vi "Ref_Num_Stopwatch_CapTest.vi"(4 "Elapsed time (seconds)":refnum<vi>, 5 "start time":refnum<vi>, 6 "stop":refnum<vi>, 7 "OK Button":refnum<vi>, 11 "Started":refnum<vi>) -> ()   [LabVIEW 2020]
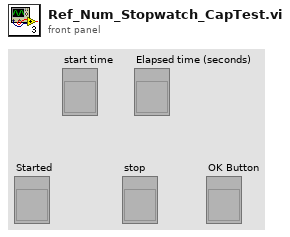
[diagram p1: front panel]
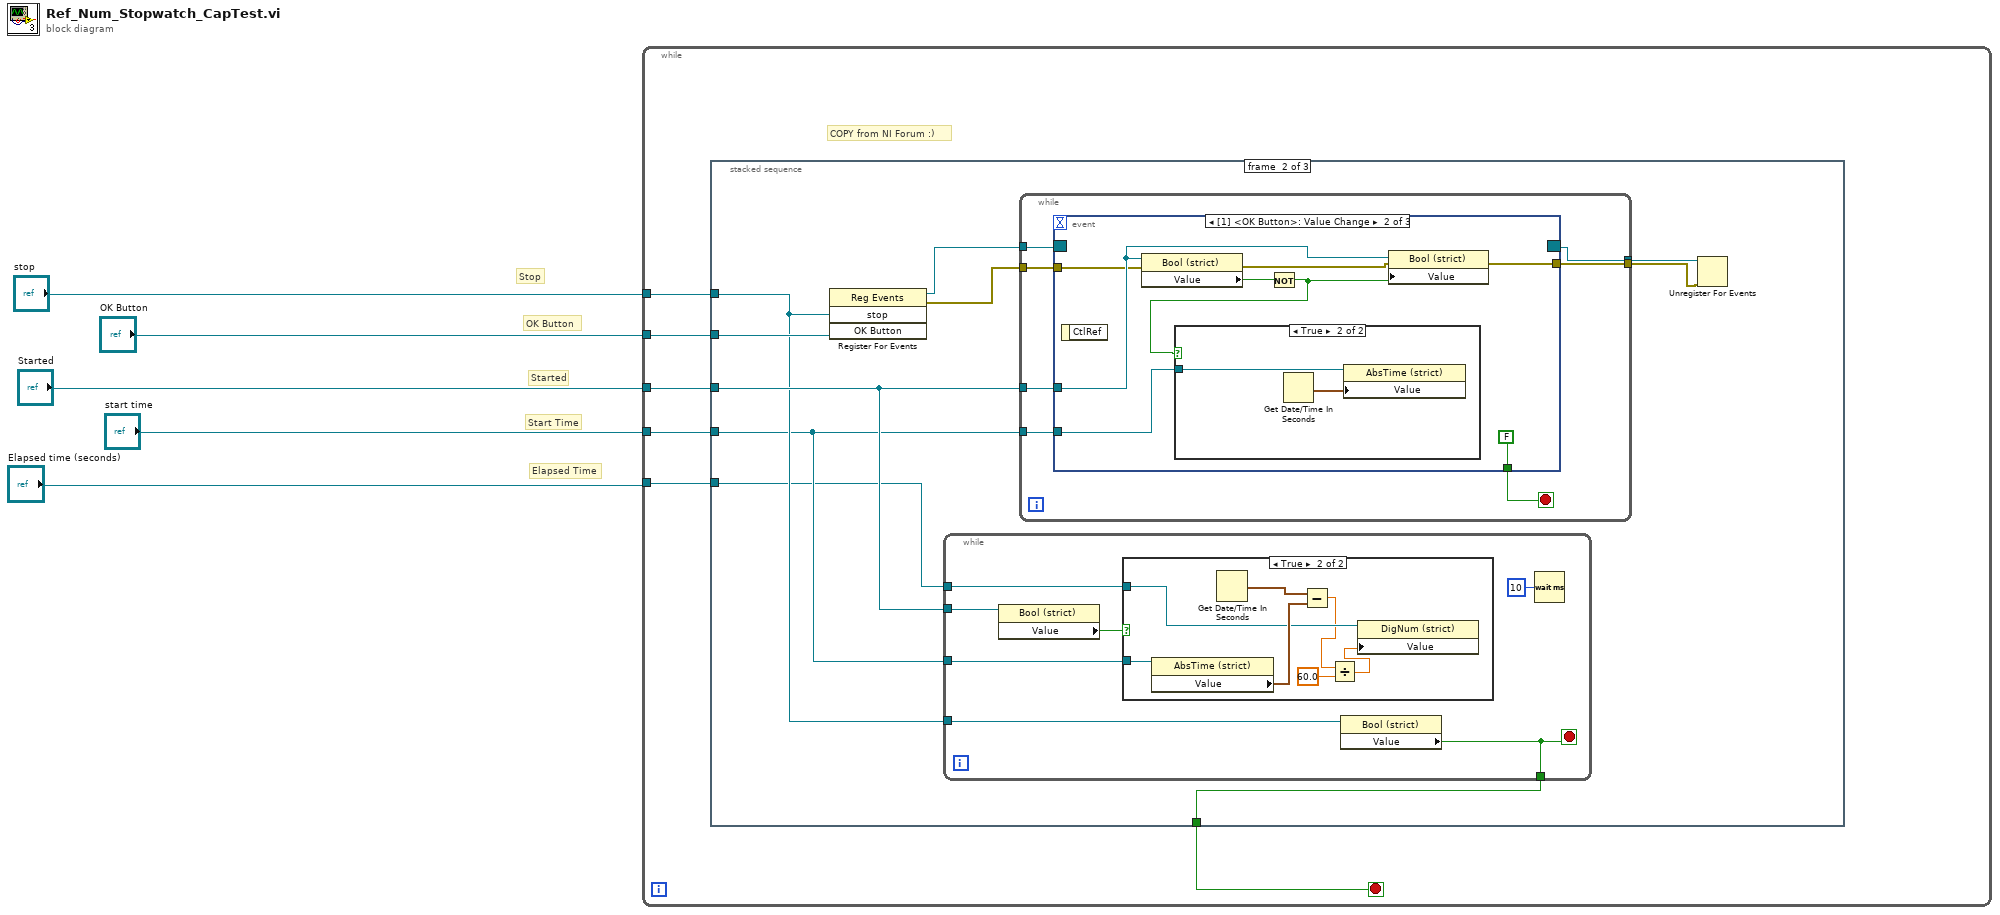
[diagram p0: block diagram]
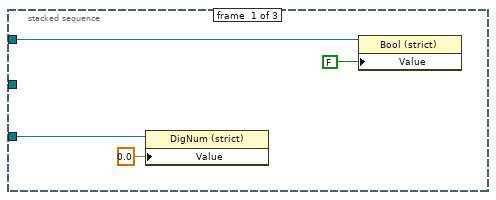
[diagram p2: hidden frame]
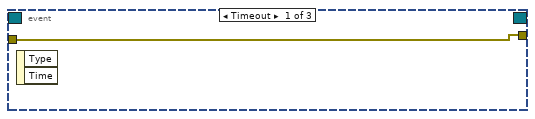
[diagram p4: hidden frame]
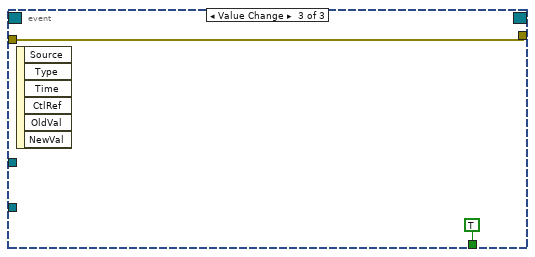
[diagram p6: hidden frame]
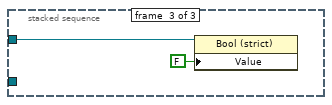
[diagram p7: hidden frame]
diagram:
  # "Elapsed Time"
  # "Start Time"
  # "Started"
  # "OK Button"
  # "Stop"
  n1 = while {
    tunnel: "Started" -> [w11]
    tunnel: "OK Button" -> [w10]
    tunnel: "Elapsed time (seconds)" -> [w9]
    tunnel: "stop" -> [w8]
    tunnel: "start time" -> [w7]
    stop <- w6 stop-if-true
    # "COPY from NI Forum :)"
    n2 = stacked-sequence {
      tunnel: [_ w25 _] -> w6
      tunnel: w11 -> [w15 w22 _]
      tunnel: w10 -> [_ w24 _]
      tunnel: w9 -> [w13 w19 _]
      tunnel: w8 -> [_ w21 w61]
      tunnel: w7 -> [_ w20 _]
      frame #0 {
        n3 = property class="DigNum (strict)"(reference=w13, "Value"=0.0 ("Elapsed time (seconds)")) -> ()  [unwired: 1 in, 2 out]
        n4 = property class="Bool (strict)"(reference=w15, "Value"=FALSE ("Started")) -> ()  [unwired: 1 in, 2 out]
      }
      frame #1 {
        n5 = register-events(w21, w24) -> (reference out=w23:refnum<event-registration>, error out=w17:errorcluster)  [unwired: 2 in]
        n6 = while {
          tunnel: [w28] -> w25
          tunnel: w22 -> [w31]
          tunnel: w21 -> [w29]
          tunnel: w20 -> [w27]
          tunnel: w19 -> [w26]
          stop <- w28 stop-if-true
          n7 = property class="Bool (strict)"(reference=w31) -> ("Value"=w30:bool)  [unwired: 1 in, 2 out]
          n8 = case shown="True" w30 {
            tunnel: w27 -> [_ w38]
            tunnel: w26 -> [_ w36]
            frame False {
              # "do nothing"
            }
            frame True {
              n9 = property class="AbsTime (strict)"(reference=w38) -> ("Value"=w37:timestamp)  [unwired: 1 in, 2 out]
              n10 = Get Date/Time In Seconds() -> (seconds since 1Jan1904=w39:timestamp)
              n11 = Subtract(x=w39, y=w37) -> (x-y=w34:dbl)
              n12 = Divide(x=w34, y=60.0) -> (x/y=w33:dbl)
              n13 = property class="DigNum (strict)"(reference=w36, "Value"=w33) -> ()  [unwired: 1 in, 2 out]
            }
          }
          n14 = property class="Bool (strict)"(reference=w29) -> ("Value"=w28:bool)  [unwired: 1 in, 2 out]
          n15 = Wait (ms)(milliseconds to wait=u32 10) -> ()  [unwired: 1 out]
        }
        n16 = while {
          tunnel: w23 -> [w45]
          tunnel: w22 -> [w44]
          tunnel: w20 -> [w43]
          tunnel: [w42] -> w18
          tunnel: w17 -> [w41]
          tunnel: [w40] -> w16
          stop <- w46 stop-if-true
          n17 = event shown="[1] <OK Button>: Value Change" {
            selector: w45 -> [_ _ _]
            dyn-events: [_ _ _] -> w42
            timeout: _ -> [_ _ _]
            tunnel: [_ FALSE TRUE] -> w46
            tunnel: w44 -> [_ w54 _]
            tunnel: w43 -> [_ w51 _]
            tunnel: w41 -> [w47 w50 w58]
            tunnel: [w47 w48 w58] -> w40
            event Timeout {
              n18 = event-data() -> ()  [unwired: 1 in, 2 out]
            }
            event Value Change {
              n19 = event-data() -> ()  [unwired: 1 in, 1 out]
              n20 = property class="Bool (strict)"(reference=w54, error in=w50) -> (error out=w49:errorcluster, "Value"=w53:bool)  [unwired: 1 out]
              n21 = Not(x=w53) -> (.not. x?=w52:bool)
              n22 = case shown="True" w52 {
                tunnel: w51 -> [_ w57]
                frame False {
                }
                frame True {
                  n23 = Get Date/Time In Seconds() -> (seconds since 1Jan1904=w56:timestamp)
                  n24 = property class="AbsTime (strict)"(reference=w57, "Value"=w56) -> ()  [unwired: 1 in, 2 out]
                }
              }
              n25 = property class="Bool (strict)"(reference=w54, error in=w49, "Value"=w52) -> (error out=w48:errorcluster)  [unwired: 1 out]
            }
            event Value Change {
              n26 = event-data() -> ()  [unwired: 1 in, 6 out]
            }
          }
        }
        n27 = Unregister For Events(event registration refnum=w18, error in=w16) -> ()  [unwired: 1 out]
      }
      frame #2 {
        n28 = property class="Bool (strict)"(reference=w61, "Value"=FALSE) -> ()  [unwired: 1 in, 2 out]
      }
    }
  }
